vi "AddMergeFile.vi"(8 "error in (no error)":errorcluster, 9 "ExistingFilePath":path, 11 "FileMerge in":refnum<class "FileMerge.lvclass">) -> (0 "error out":errorcluster, 3 "FileMerge out":refnum<class "FileMerge.lvclass">)   [LabVIEW 2019, in "FileMerge.lvclass"]
uses:
  FileMerge.lvclass
  ExistingFileMgr/ExistingFileMgr.lvclass
  FileMerge.lvclass/FileMerge.ctl
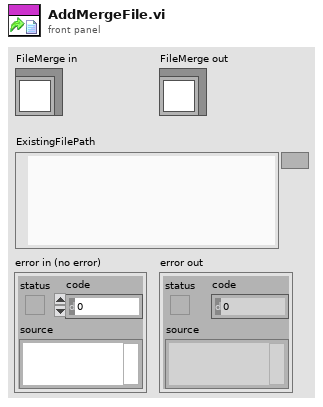
[diagram p1: front panel]
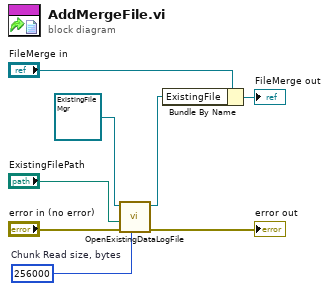
[diagram p0: block diagram]
diagram:
  w1 = 256000  # Chunk Read size, bytes
  n1 = call "OpenExistingDataLogFile.vi"("Chunk Read size, bytes"=w1, "error in (no error)"="error in (no error)", "ExistingFilePath"="ExistingFilePath", "ExistingFileMgr in"=refnum<class "ExistingFileMgr.lvclass"> refnum) -> ("error out"=→"error out":errorcluster, "ExistingFileMgr out"=w5:refnum<class "ExistingFileMgr.lvclass">)  [unwired: 6 in]
  n2 = Bundle By Name(cluster="FileMerge in", "ExistingFile"=w5) -> (→"FileMerge out":refnum<class "FileMerge.lvclass">)
